vi "子VI-缺陷面积筛选.vi"(9 "计入分层缺陷的面积阈值":i32, 11 "分层测量结果":dbl[][](array[numeric])) -> (2 "初始化的数组":dbl[][](array[numeric]), 3 "去掉的面积累计":dbl)   [LabVIEW 2018]
panel:
  out "数值":i32
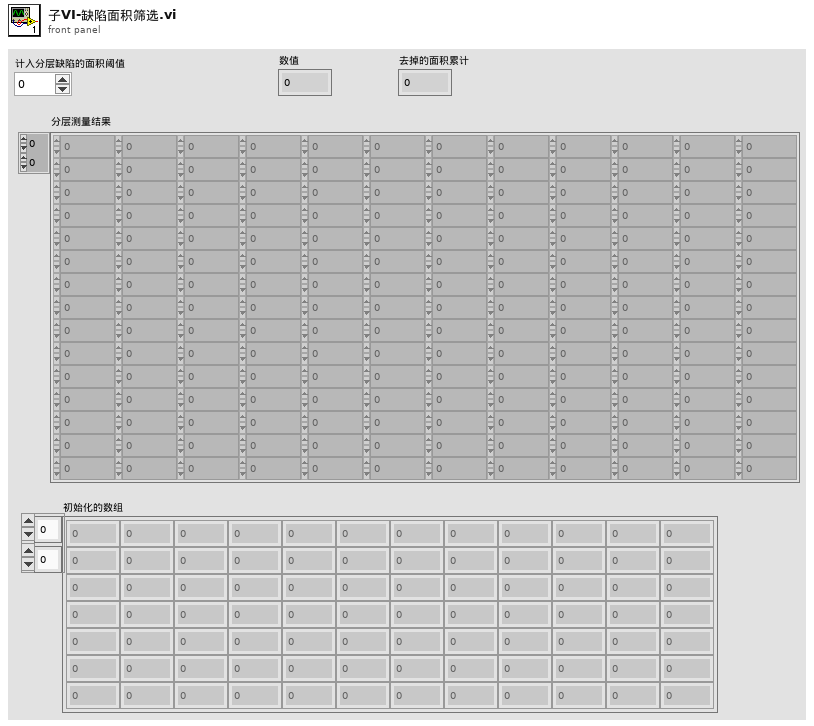
[diagram p1: front panel]
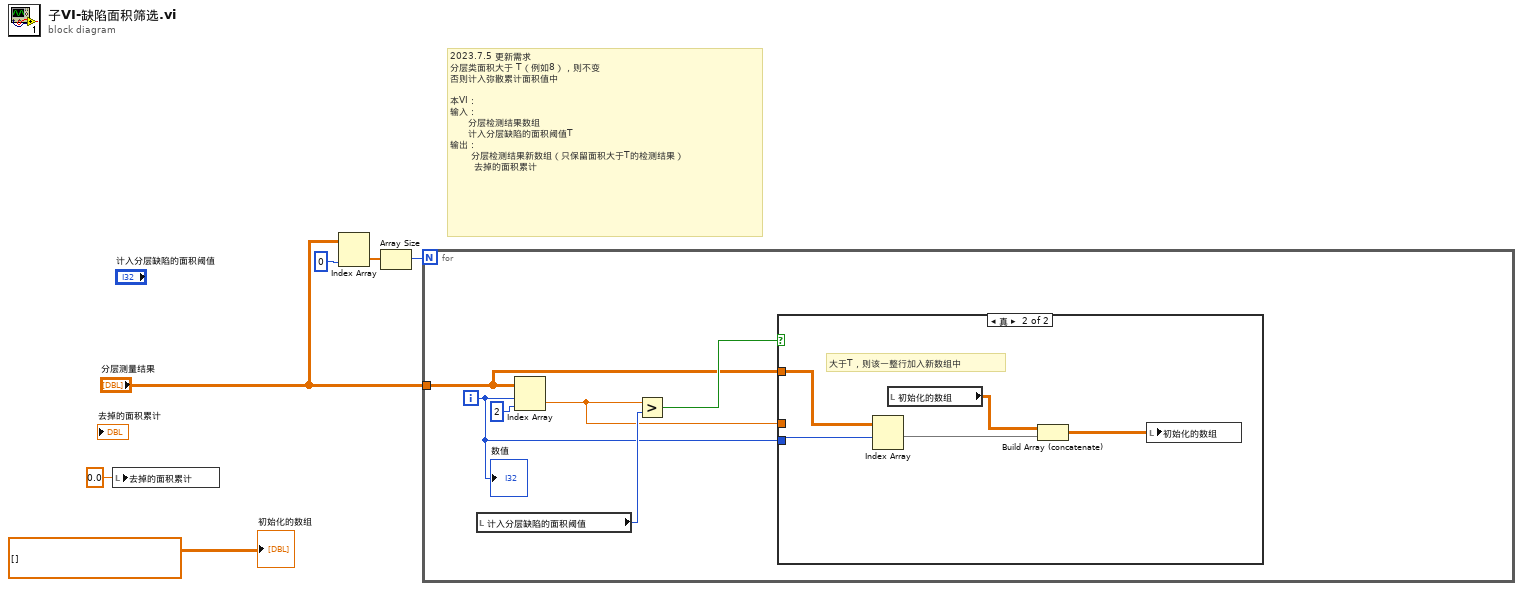
[diagram p0: block diagram]
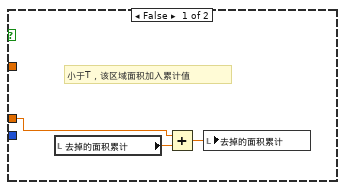
[diagram p2: hidden frame]
diagram:
  # "2023.7.5 更新需求\n分层类面积大于 T（例如8），则不变\n否则计入弥散累计面积值中\n\n本VI：\n输入：\n      分层检测结果数组\n      计入分层缺陷的面积阈值T\n输出：\n       分层检测结果新数组（只保留面积大于T的检测结果）\n        去掉的面积累计"
  n1 = local write "去掉的面积累计"(0.0 ("去掉的面积累计")) -> ()
  n2 = Index Array(array="分层测量结果", index (col)=0 ("禁用的索引 (列)")) -> (element=w4:dbl[])  [unwired: 1 in]
  n3 = Array Size(array=w4) -> (size(s)=w5:i32)
  n4 = for {
    N: w5 -> [_]
    tunnel: "分层测量结果" -> [w7]
    i -> [w8]
    n5 = local read "计入分层缺陷的面积阈值"() -> (w11:i32)
    n6 = Index Array(array=w7, index (row)=w8, index (col)=2 ("索引 (列)")) -> (element=w9:dbl)
    n7 = Greater?(x=w9, y=w11) -> (0:w10:bool)
    n8 = case shown="真" w10 {
      tunnel: w9 -> [w13 _]
      tunnel: w8 -> [_ w16]
      tunnel: w7 -> [_ w20]
      frame False {
        # "小于T，该区域面积加入累计值"
        n9 = local read "去掉的面积累计"() -> (w14:dbl)
        n10 = Add(x=w13, y=w14) -> (x+y=w15:dbl)
        n11 = local write "去掉的面积累计"(w15) -> ()
      }
      frame True {
        # "大于T，则该一整行加入新数组中"
        n12 = Index Array(array=w20, index (row)=w16) -> (element=w19:dbl[])  [unwired: 1 in]
        n13 = local read "初始化的数组"() -> (w18:dbl[][])
        n14 = Build Array (concatenate)(w18, w19) -> (w17:dbl[][])
        n15 = local write "初始化的数组"(w17) -> ()
      }
    }
    "数值" <- w8
  }
  "初始化的数组" <- dbl[][] [] ("初始化的数组")
